vi "AVG_TRACE.vi"(0 "Session In":refnum<visa-resource-name>="GPIB0::16::INSTR", 1 "Timeout":u32=3000, 5 "AVG Count":i32=16, 11 "error in":errorcluster {"code" format="%.0x"}, 12 "Trace Type (0: Clear Write)":i32(ring) items=["Clear Write", "Average", "Maximum Hold", "Minimum Hold"], 13 "AVG Restart (T)":bool, 14 "Send OPC? (T)":bool) -> (4 "Session Out":refnum<visa-resource-name>, 15 "error out":errorcluster {"code" format="%.0x"})   [LabVIEW 2018]
doc: "Launches the Instrument I/O Assistant, which you can use to communicate with message-based instruments and graphically parse the response. For example you can communicate with an instrument that uses a serial, Ethernet, or GPIB interface."
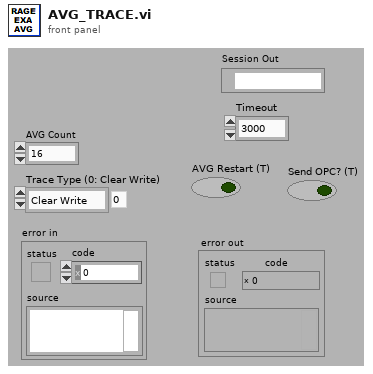
[diagram p1: front panel]
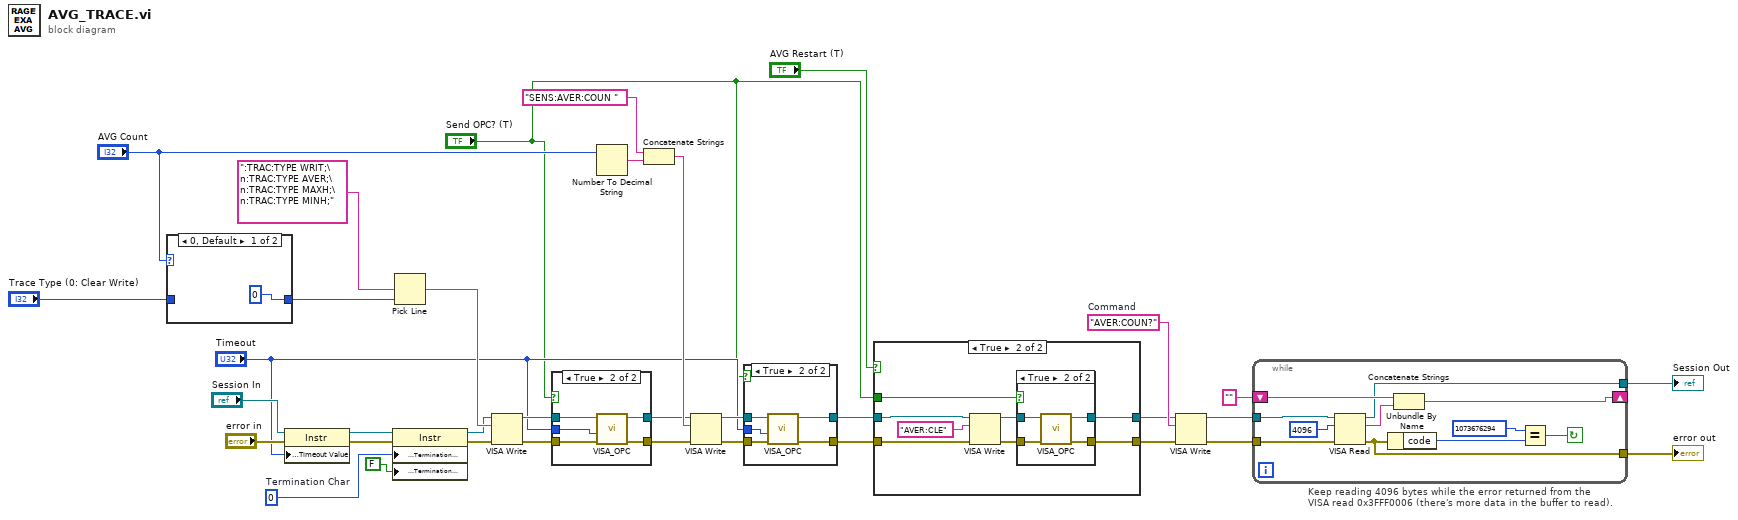
[diagram p0: block diagram]
diagram:
  w19 = "AVER:COUN?"  # Command
  w32 = u8 0  # Termination Char
  # "Keep reading 4096 bytes while the error returned from the\nVISA read 0x3FFF0006 (there's more data in the buffer to read)."
  n1 = case shown="0, Default" "AVG Count" {
    tunnel: [0 ("AVG Count") w37] -> w22
    tunnel: "Trace Type (0: Clear Write)" -> [_ w37]
    frame 0, Default {
    }
    frame 1.. {
    }
  }
  n2 = property class="Instr"(reference="Session In", error in="error in", "General Settings:Timeout Value"="Timeout") -> (reference out=w31:refnum<visa-resource-name>, error out=w33:errorcluster)
  n3 = property class="Instr"(reference=w31, error in=w33, "Message Based Settings:Termination Character"=w32, "Message Based Settings:Termination Character Enable"=FALSE ("enable")) -> (reference out=w14:refnum<visa-resource-name>, error out=w13:errorcluster)
  n4 = Pick Line(multi-line string=":TRAC:TYPE WRIT;\n:TRAC:TYPE AVER;\n:TRAC:TYPE MAXH;\n:TRAC:TYPE MINH;", line index=w22) -> (output string=w24:string)  [unwired: 1 in]
  n5 = VISA Write(VISA resource name=w14, write buffer=w24, error in (no error)=w13) -> (VISA resource name out=w7:refnum<visa-resource-name>, error out=w10:errorcluster)  [unwired: 1 out]
  n6 = case shown="True" "Send OPC? (T)" {
    tunnel: w10 -> [w39 w44]
    tunnel: [w39 w43] -> w9
    tunnel: [w38 w42] -> w8
    tunnel: w7 -> [w38 w41]
    tunnel: "Timeout" -> [_ w40]
    frame False {
    }
    frame True {
      n7 = call "VISA_OPC.vi"("error in"=w44, "Timeout"=w40, "Session In"=w41) -> ("error out"=w43:errorcluster, "Session Out"=w42:refnum<visa-resource-name>)  [unwired: 6 in, 1 out]
    }
  }
  n8 = Number To Decimal String(number="AVG Count") -> (decimal integer string=w29:string)  [unwired: 1 out]
  n9 = Concatenate Strings("SENS:AVER:COUN " ("staticText"), w29) -> (w27:string)
  n10 = VISA Write(VISA resource name=w8, write buffer=w27, error in (no error)=w9) -> (VISA resource name out=w5:refnum<visa-resource-name>, error out=w6:errorcluster)  [unwired: 1 out]
  n11 = case shown="True" "Send OPC? (T)" {
    tunnel: w6 -> [w45 w51]
    tunnel: w5 -> [w46 w50]
    tunnel: "Timeout" -> [_ w49]
    tunnel: [w45 w48] -> w3
    tunnel: [w46 w47] -> w2
    frame False {
    }
    frame True {
      n12 = call "VISA_OPC.vi"("error in"=w51, "Timeout"=w49, "Session In"=w50) -> ("error out"=w48:errorcluster, "Session Out"=w47:refnum<visa-resource-name>)  [unwired: 6 in, 1 out]
    }
  }
  n13 = case shown="True" "AVG Restart (T)" {
    tunnel: w3 -> [w52 w61]
    tunnel: [w52 w58] -> w18
    tunnel: w2 -> [w53 w59]
    tunnel: [w53 w55] -> w16
    tunnel: "Send OPC? (T)" -> [_ w54]
    frame False {
    }
    frame True {
      n14 = VISA Write(VISA resource name=w59, write buffer="AVER:CLE" ("StaticText"), error in (no error)=w61) -> (VISA resource name out=w56:refnum<visa-resource-name>, error out=w57:errorcluster)  [unwired: 1 out]
      n15 = case shown="True" w54 {
        tunnel: [w62 w67] -> w58
        tunnel: w57 -> [w62 w66]
        tunnel: w56 -> [w63 w65]
        tunnel: [w63 w64] -> w55
        frame False {
        }
        frame True {
          n16 = call "VISA_OPC.vi"("error in"=w66, "Session In"=w65) -> ("error out"=w67:errorcluster, "Session Out"=w64:refnum<visa-resource-name>)  [unwired: 7 in, 1 out]
        }
      }
    }
  }
  n17 = VISA Write(VISA resource name=w16, write buffer=w19, error in (no error)=w18) -> (VISA resource name out=w15:refnum<visa-resource-name>, error out=w17:errorcluster)  [unwired: 1 out]
  n18 = while {
    tunnel: w15 -> [w75]
    shift-right: [w69] -> _
    shift-left: "" -> [w74]
    tunnel: w17 -> [w72]
    tunnel: [w71] -> w11
    tunnel: [w68] -> w12
    stop <- w70 continue-if-true
    n19 = VISA Read(VISA resource name=w75, byte count=u32 4096 ("byte count (0)"), error in (no error)=w72) -> (VISA resource name out=w68:refnum<visa-resource-name>, read buffer=w73:string, error out=w71:errorcluster)  [unwired: 1 out]
    n20 = Unbundle By Name(w71) -> ("code"=w77:i32)
    n21 = Concatenate Strings(w74, w73) -> (w69:string)
    n22 = Equal?(x=1073676294, y=w77) -> (x = y?=w70:bool)
  }
  "error out" <- w11
  "Session Out" <- w12
